vi "Pre Launch Init.vi"(11 "VoiceControl in":refnum<class "Voice.lvclass"> caption="操作者输入") -> (0 "error out":errorcluster caption="错误输出", 3 "VoiceControl out":refnum<class "Voice.lvclass"> caption="操作者输出")   [LabVIEW 2014, in "Voice.lvlib" / "Voice.lvclass"]
doc: "(<B>Filename</B>: Actor Framework.lvlib:Actor.lvclass:Pre Launch Init.vi)\n\nDefines behavior that occurs after the Launch Nested Actor method is invoked but before the actor's Actor Core method begins running.\n\nBy default, this method does nothing. A descendant class may override it to define behavior."
uses:
  Voice.lvclass
  Voice.lvclass/Voice.ctl
  <vilib>/ActorFramework/Actor/Actor.lvclass
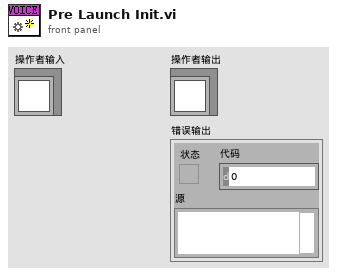
[diagram p1: front panel]
types:
  T1 = cluster{"Stop":refnum<user-event>, "Text":refnum<user-event>, "Connected":refnum<user-event>}
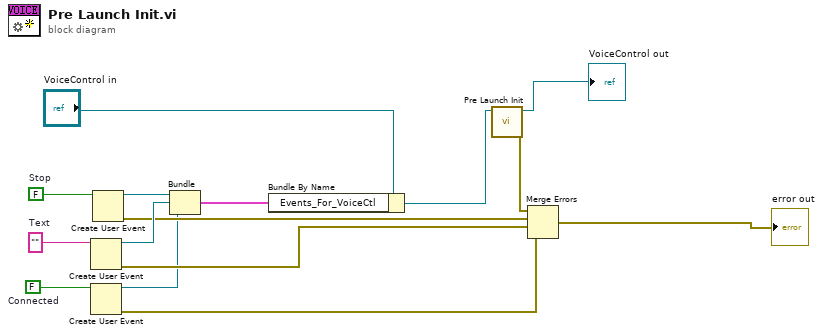
[diagram p0: block diagram]
diagram:
  w8 = FALSE  # Connected
  w14 = FALSE  # Stop
  w15 = ""  # Text
  n1 = Create User Event(user event datatype=w15) -> (user event=w12:refnum<user-event>, error out=w9:errorcluster)  [unwired: 1 in]
  n2 = Create User Event(user event datatype=w8) -> (user event=w6:refnum<user-event>, error out=w7:errorcluster)  [unwired: 1 in]
  n3 = Create User Event(user event datatype=w14) -> (user event=w13:refnum<user-event>, error out=w10:errorcluster)  [unwired: 1 in]
  n4 = Bundle("Stop"=w13, "Text"=w12, "Connected"=w6) -> (w11:T1)  [unwired: 1 in]
  n5 = Bundle By Name(cluster="VoiceControl in", "Events_For_VoiceCtl"=w11) -> (w4:refnum<class "Voice.lvclass">)
  n6 = call-parent "Pre Launch Init.vi"("Actor in"=w4) -> ("error out"=w5:errorcluster, "Actor out"=→"VoiceControl out":refnum<class "Voice.lvclass">)  [unwired: 9 in]
  n7 = Merge Errors(w5, w10, w9, w7) -> (→"error out":errorcluster)
